vi "_Sample Generator.vi"() -> ()   [LabVIEW 2013]
panel:
  out "VISA Refnum out":refnum<visa-resource-name>
  out "concatenated string":string
  in  "elemszam":u16
  out "error out":errorcluster
  in  "VISA resource name":refnum<visa-resource-name>
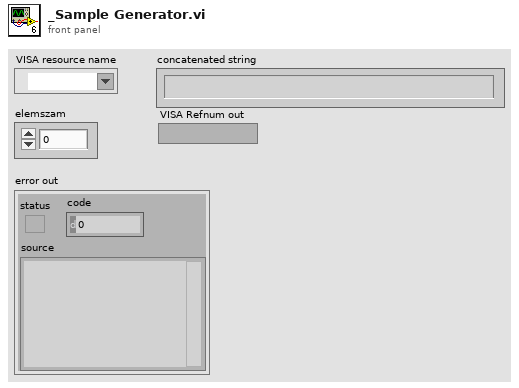
[diagram p1: front panel]
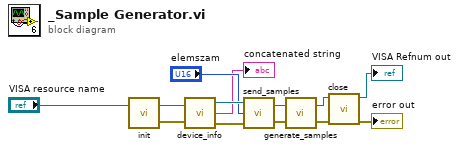
[diagram p0: block diagram]
diagram:
  n1 = call "init.vi"("VISA Refnum in"="VISA resource name") -> ("error out"=w11:errorcluster, "VISA Refnum out"=w12:refnum<visa-resource-name>)  [unwired: 1 in]
  n2 = call "device_info.vi"("VISA Refnum in"=w12, "error in (no error)"=w11) -> ("VISA Refnum out"=w10:refnum<visa-resource-name>, "concatenated string"=→"concatenated string":string, "error out"=w9:errorcluster)
  n3 = call "send_samples.vi"("error in (no error)"=w9, "elemszam"="elemszam", "VISA Refnum in"=w10) -> ("error out"=w3:errorcluster, "VISA Refnum out"=w4:refnum<visa-resource-name>)
  n4 = call "generate_samples.vi"("error in (no error)"=w3, "VISA Refnum in"=w4) -> ("error out"=w1:errorcluster, "VISA Refnum out"=w2:refnum<visa-resource-name>)
  n5 = call "close.vi"("error in (no error)"=w1, "VISA resource name"=w2) -> ("error out"=→"error out":errorcluster, "VISA resource name out"=→"VISA Refnum out":refnum<visa-resource-name>)  [unwired: 4 in]
